vi "serial_open.vi"(8 "error in":errorcluster, 11 "VISA Refnum in":refnum<visa-resource-name>="COM1") -> (0 "error out":errorcluster, 3 "VISA Refnum out":refnum<visa-resource-name>)   [LabVIEW 2019]
uses:
  <vilib>/Instr/_visa.llb/VISA Configure Serial Port (Instr).vi
  C:/Program Files (x86)/National Instruments/LabVIEW 2019/examples/Instrument IO/Serial/support/Serial - Settings.ctl
  C:/Program Files (x86)/National Instruments/LabVIEW 2019/examples/Instrument IO/Serial/support/Serial - ASCII Characters.ctl
  C:/Program Files (x86)/National Instruments/LabVIEW 2019/examples/Instrument IO/Serial/support/Serial - XON-XOFF Characters.ctl
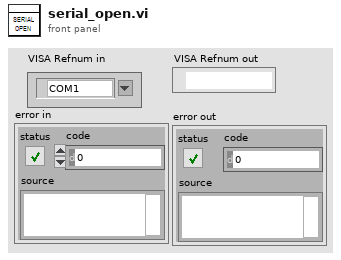
[diagram p1: front panel]
types:
  T1 = typedef "Serial - XON-XOFF Characters.ctl" = cluster{"XON":T2, "XOFF":T2}
  T2 = typedef "Serial - ASCII Characters.ctl" = enum16{"NUL", "SOH", "STX", "ETX", "EOT", "ENQ", "ACK", "BEL", "BS", "HT", "LF", "VT", "FF", "CR", "SO", "SI", "DLE", "DC1", "DC2", "DC3", "DC4", "NAK", "SYN", "ETB", "CAN", "EM", "SUB", "ESC", "FS", "GS", "RS", "US", "SP", "!", "\"", "#", "$", "%", "&", "'", "(", ")", "*", "+", ",", "- (-)", ".", "/", "0", "1", "2", "3", "4", "5", "6", "7", "8", "9", ":", ";", "<", "=", ">", "?", "@", "A", "B", "C", "D", "E", "F", "G", "H", "I", "J", "K", "L", "M", "N", "O", "P", "Q", "R", "S", "T", "U", "V", "W", "X", "Y", "Z", "[", "\\", "]", "^", "_", "`", "a", "b", "c", "d", "e", "f", "g", "h", "i", "j", "k", "l", "m", "n", "o", "p", "q", "r", "s", "t", "u", "v", "w", "x", "y", "z", "{", "|", "}", "~"}
  T3 = typedef "Serial - Settings.ctl" = cluster{"baud rate":u32, "data bits":u16, "parity":enum16{"None", "Odd", "Even", "Mark", "Space"}, "stop bits":u16, "flow control":u16}
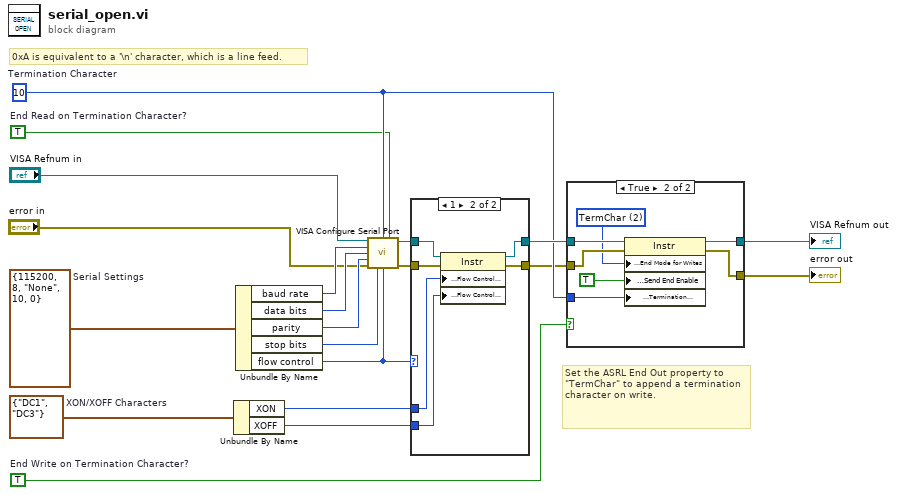
[diagram p0: block diagram]
diagram:
  w18 = TRUE  # End Write on Termination Character?
  w3 = T1 {"XON"=enum."DC1", "XOFF"=enum."DC3"}  # XON/XOFF Characters
  w10 = T3 {"baud rate"=115200, "data bits"=8, "parity"=enum."None", "stop bits"=10, "flow control"=0}  # Serial Settings
  w19 = u8 10  # Termination Character
  w11 = TRUE  # End Read on Termination Character?
  # "0xA is equivalent to a '\\n' character, which is a line feed."
  # "Set the ASRL End Out property to \"TermChar\" to append a termination character on write."
  n1 = Unbundle By Name(w3) -> ("XON"=w13:T2, "XOFF"=w14:T2)
  n2 = Unbundle By Name(w10) -> ("baud rate"=w9:u32, "data bits"=w8:u16, "parity"=w7:enum16{"None", "Odd", "Even", "Mark", "Space"}, "stop bits"=w6:u16, "flow control"=w12:u16)
  n3 = call-poly "VISA Configure Serial Port"("VISA resource name"="VISA Refnum in", "termination char\n(0xA = '\\n' = LF)"=w19, "Enable Termination\nChar (T)"=w11, "baud rate (9600)"=w9, "data bits (8)"=w8, "parity (0:none)"=w7, "error in (no error)"="error in", "stop bits (10: 1 bit)"=w6, "flow control (0:none)"=w12) -> ("VISA resource name out"=w5:refnum<visa-resource-name>, "error out"=w4:errorcluster)  [unwired: 1 in, 4 out]
  n4 = case shown="1" w12 {
    tunnel: [w21 w28] -> w15
    tunnel: [w22 w27] -> w20
    tunnel: w4 -> [w21 w26]
    tunnel: w5 -> [w22 w25]
    tunnel: w13 -> [_ w24]
    tunnel: w14 -> [_ w23]
    frame Default {
    }
    frame 1 {
      n5 = property class="Instr"(reference=w25, error in=w26, "Serial Settings:Flow Control XON Character"=w24, "Serial Settings:Flow Control XOFF Character"=w23) -> (reference out=w27:refnum<visa-resource-name>, error out=w28:errorcluster)
    }
  }
  n6 = case shown="True" w18 {
    tunnel: w20 -> [w29 w37]
    tunnel: w15 -> [w30 w36]
    tunnel: [w29 w35] -> w17
    tunnel: [w30 w34] -> w16
    tunnel: w19 -> [_ w32]
    frame False {
    }
    frame True {
      w33 = u16 2 items=["None", "LastBit", "TermChar", "Break"] ("Serial Settings:Serial End Mode for Writes")
      n7 = property class="Instr"(reference=w37, error in=w36, "Serial Settings:End Mode for Writes"=w33, "Message Based Settings:Send End Enable"=TRUE, "Message Based Settings:Termination Character"=w32) -> (reference out=w35:refnum<visa-resource-name>, error out=w34:errorcluster)
    }
  }
  "VISA Refnum out" <- w17
  "error out" <- w16
